vi "Reset Message Queue.vi"(8 "error in (no error)":errorcluster, 11 "Message Queue":refnum<queue>) -> (0 "error out":errorcluster, 3 "dup Message Queue":refnum<queue>)   [LabVIEW 2024, in "Message Queue.lvlib"]
doc: "Removes all the message from message queue."
uses:
  Message Queue.lvlib
  Message Cluster.ctl
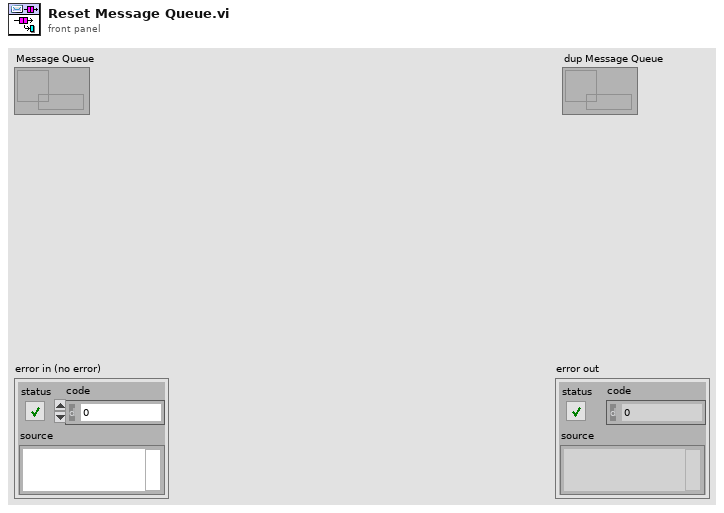
[diagram p1: front panel]
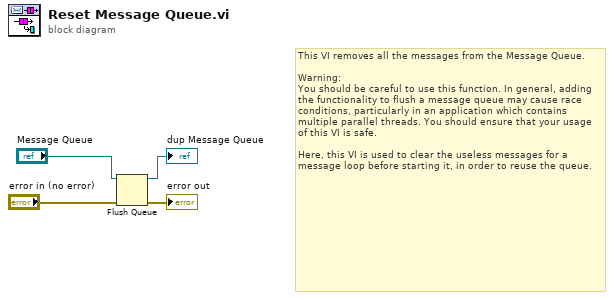
[diagram p0: block diagram]
diagram:
  # "This VI removes all the messages from the Message Queue.\n\nWarning:\nYou should be careful to use this function. In general, adding the functionality to flush a message queue may cause race conditions, particularly in an application which contains multiple parallel threads. You should ensure that your usage of this VI is safe.\n\nHere, this VI is used to clear the useless messages for a message loop before starting it, in order to reuse the queue."
  n1 = Flush Queue(queue="Message Queue", error in (no error)="error in (no error)") -> (queue out=→"dup Message Queue":refnum<queue>, error out=→"error out":errorcluster)  [unwired: 1 out]
